vi "onCreated.vi"(8 "error in (no error)":errorcluster, 11 "Camera.Simulated":refnum<class "Camera.Simulated.lvclass">) -> (0 "error out":errorcluster, 3 "Camera.Simulated out":refnum<class "Camera.Simulated.lvclass">)   [LabVIEW 2015, in "Camera.Simulated.lvclass"]
doc: "JKI State Machine Objects (SMO) 1.0.4.18\nJKI - JKI\nCopyright (c) 2016, JKI"
uses:
  Camera.Simulated.lvclass
  Configuration--CLuster.ctl
  <vilib>/picture/picture.llb/imagedata.ctl
  <userlib>/_OpenG.lib/file/file.llb/File Exists - Scalar__ogtk.vi
  <userlib>/_OpenG.lib/file/file.llb/Valid Path - Traditional__ogtk.vi
  Camera/Camera.lvclass
  CircularBuffer.ImageData/CircularBuffer.ImageData.lvclass
  <vilib>/JKI/JKI SMO/SMO/SMO.lvclass
  <vilib>/Utility/config.llb/NI_LVConfig.lvlib
panel:
  # "For instructions on how to use the JKI State Machine Objects, examples and video tutorials, visit:\nhttp://jki.net/state-machine-objects/\n\nJKI State Machine Objects™\nhttp://jki.net/state-machine-objects/\nCopyright (C) 2005-2015, JKI <info@jki.net>\nALL RIGHTS RESERVED"
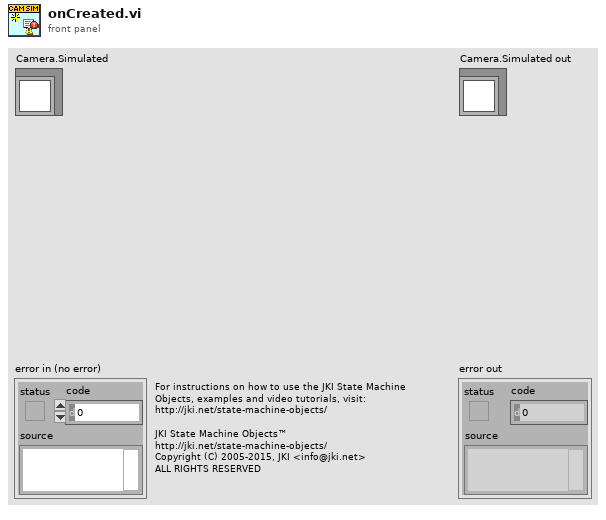
[diagram p1: front panel]
types:
  T1 = typedef "Camera.Simulated.lvclass/Configuration--CLuster.ctl" = cluster{"Simulated Images Folder":path, "filetype":string}
  T2 = typedef "NI_LVConfig.lvlib/Config Data RefNum.ctl" = refnum<k1>
  T3 = typedef "imagedata.ctl" = cluster{"image type":i32, "image depth":i32, "image":u8[], "mask":u8[], "colors":u32[], "Rectangle":cluster{"left":i16, "top":i16, "right":i16, "bottom":i16}}
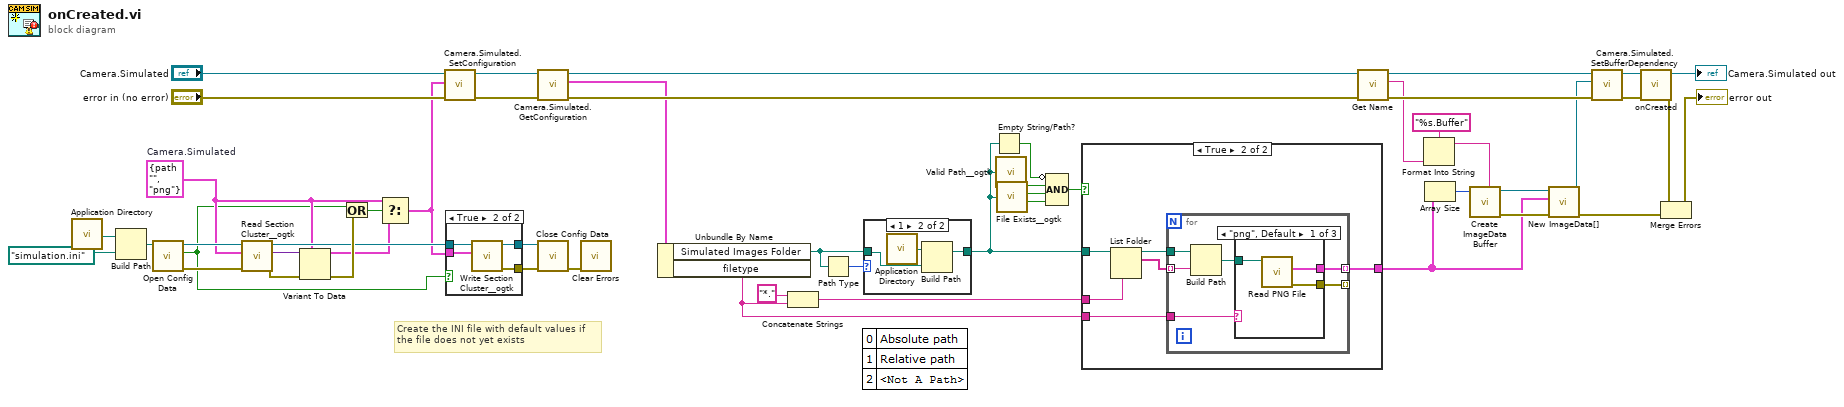
[diagram p0: block diagram]
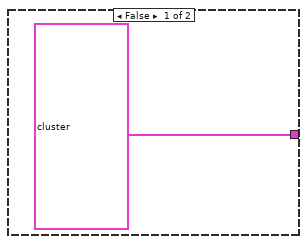
[diagram p4: hidden frame]
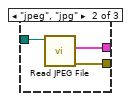
[diagram p5: hidden frame]
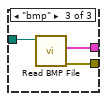
[diagram p6: hidden frame]
diagram:
  w3 = T1 {"Simulated Images Folder"=path "", "filetype"="png"}  # Camera.Simulated
  # "Create the INI file with default values if\nthe file does not yet exists"
  n1 = call <vilib>:"Application Directory.vi"() -> ("Application Directory"=w30:path)
  n2 = Build Path(base path=w30, name or relative path=path "simulation.ini") -> (appended path=w4:path)
  n3 = call <vilib>:"Open Config Data.vi"("configuration file path"=w4) -> ("error out"=w8:errorcluster, "file created?"=w1:bool, "refnum"=w6:T2)  [unwired: 8 in]
  n4 = call <userlib>:"Read Section Cluster__ogtk.vi"("error in (no error)"=w8, "Section Formatted Cluster Type"=w3, "refnum"=w6) -> ("error out"=w13:errorcluster, "Section Formatted Cluster"=w7:variant, "dup refnum"=w9:T2)  [unwired: 4 in, 2 out]
  n5 = Variant To Data(error in=w13, type=w3, Variant=w7) -> (data=w5:T1, error out=w14:errorcluster)
  n6 = Or(x=w1, y=w14) -> (x .or. y?=w15:bool)
  n7 = Select(t=w3, s=w15, f=w5) -> (s? t:f=w2:T1)
  n8 = call "Camera.Simulated.SetConfiguration.vi"("error in (no error)"="error in (no error)", "Configuration"=w2, "Camera.Simulated"="Camera.Simulated") -> ("error out"=w27:errorcluster, "Camera.Simulated"=w25:refnum<class "Camera.Simulated.lvclass">)  [unwired: 7 in]
  n9 = case shown="True" w1 {
    tunnel: w9 -> [w52 w56]
    tunnel: w2 -> [_ w55]
    tunnel: [_ w54] -> w10
    tunnel: [w52 w53] -> w11
    frame False {
    }
    frame True {
      n10 = call <userlib>:"Write Section Cluster__ogtk.vi"("Section Formatted Cluster"=w55, "refnum"=w56) -> ("error out"=w54:errorcluster, "dup refnum"=w53:T2)  [unwired: 8 in]
    }
  }
  n11 = call "Camera.Simulated.GetConfiguration.vi"("error in (no error)"=w27, "Camera.Simulated"=w25) -> ("error out"=w26:errorcluster, "Configuration"=w24:T1, "Camera.Simulated"=w28:refnum<class "Camera.Simulated.lvclass">)  [unwired: 7 in]
  n12 = call <vilib>:"Close Config Data.vi"("error in (no error)"=w10, "refnum"=w11) -> ("error out"=w12:errorcluster)  [unwired: 8 in, 1 out]
  n13 = call <vilib>:"Clear Errors.vi"("error in (no error)"=w12) -> ()  [unwired: 5 in, 2 out]
  n14 = Unbundle By Name(w24) -> ("Simulated Images Folder"=w17:path, "filetype"=w19:string)
  n15 = Concatenate Strings("*." ("pattern"), w19) -> (w20:string)
  n16 = Path Type(1:w17) -> (0:w18:i16)
  n17 = case shown="1" w18 {
    tunnel: w17 -> [w57 w58]
    tunnel: [w57 w60] -> w16
    frame 0, Default {
    }
    frame 1 {
      n18 = call <vilib>:"Application Directory.vi"() -> ("Application Directory"=w59:path)
      n19 = Build Path(base path=w59, name or relative path=w58) -> (appended path=w60:path)
    }
  }
  n20 = Empty String/Path?(string/path=w16) -> (empty?=w34:bool)
  n21 = call-poly <userlib>:"Valid Path__ogtk.vi"("path"=w16) -> ("valid"=w35:bool)
  n22 = call-poly <userlib>:"File Exists__ogtk.vi"("file path"=w16) -> ("is directory"=w36:bool, "exists"=w37:bool)  [unwired: 6 in]
  n23 = Compound Arithmetic op=AND(invert w34, w35, w36, w37) -> (w31:bool)
  n24 = case shown="True" w31 {
    tunnel: w16 -> [_ w66]
    tunnel: [T3[] data[49993B] ("Array") w64] -> w33
    tunnel: w20 -> [_ w63]
    tunnel: w19 -> [_ w62]
    frame False {
    }
    frame True {
      n25 = List Folder(path=w66, pattern=w63) -> (path out=w67:path, filenames=w65:string[])  [unwired: 2 in, 2 out]
      n26 = for {
        tunnel: w67 -> [w73]
        tunnel: w65 -> [w71] mode=indexing
        tunnel: [w70] -> w64 mode=indexing
        tunnel: [w69] -> _ mode=indexing
        tunnel: w62 -> [w68]
        n27 = Build Path(base path=w73, name or relative path=w71) -> (appended path=w72:path)
        n28 = case shown="\"png\", Default" w68 {
          tunnel: w72 -> [w76 w79 w82]
          tunnel: [w75 w78 w81] -> w70
          tunnel: [w74 w77 w80] -> w69
          frame "png", Default {
            n29 = call <vilib>:"Read PNG File.vi"("path to PNG file"=w76) -> ("error out"=w74:errorcluster, "image data"=w75:T3)  [unwired: 8 in, 1 out]
          }
          frame "jpeg", "jpg" {
            n30 = call <vilib>:"Read JPEG File.vi"("path to JPEG file"=w79) -> ("error out"=w77:errorcluster, "image data"=w78:T3)  [unwired: 8 in, 1 out]
          }
          frame "bmp" {
            n31 = call <vilib>:"Read BMP File.vi"("path to BMP file"=w82) -> ("error out"=w80:errorcluster, "image data"=w81:T3)  [unwired: 8 in, 1 out]
          }
        }
      }
    }
  }
  n32 = call <vilib>:"Get Name.vi"("error in (no error)"=w26, "SMO"=w28) -> ("error out"=w48:errorcluster, "Name"=w32:string, "SMO out"=w49:refnum<class "Camera.Simulated.lvclass">)  [unwired: 7 in]
  n33 = Format Into String(format string="%s.Buffer", w32) -> (resulting string=w47:string)  [unwired: 2 in, 1 out]
  n34 = Array Size(array=w33) -> (size(s)=w40:i32)
  n35 = call "Create ImageData Buffer.vi"("Buffer Name"=w47, "BufferSize"=w40) -> ("error out"=w39:errorcluster, "CircularBuffer.ImageData out"=w42:refnum<class "CircularBuffer.ImageData.lvclass">)  [unwired: 7 in, 1 out]
  n36 = call "New ImageData[].vi"("error in (no error)"=w39, "ImageData[]"=w33, "CircularBuffer.ImageData"=w42) -> ("error out"=w38:errorcluster, "CircularBuffer.ImageData out"=w41:refnum<class "CircularBuffer.ImageData.lvclass">)  [unwired: 6 in, 1 out]
  n37 = call "Camera.Simulated.SetBufferDependency.vi"("error in (no error)"=w48, "CircularBuffer.ImageData"=w41, "Camera.Simulated"=w49) -> ("error out"=w50:errorcluster, "Camera.Simulated"=w51:refnum<class "Camera.Simulated.lvclass">)  [unwired: 7 in]
  n38 = call-parent "onCreated.vi"("error in (no error)"=w50, "Camera"=w51) -> ("error out"=w45:errorcluster, "Camera"=→"Camera.Simulated out":refnum<class "Camera.Simulated.lvclass">)  [unwired: 8 in]
  n39 = Merge Errors(w45, w38) -> (→"error out":errorcluster)
